vi "ReadXML_SRSI.vi"(8 "error in (no error)":errorcluster, 11 "XML File Path":path) -> (0 "error out":errorcluster, 2 "SRSI Parameters":T1={"sensitivity"=0.11032028469750889, "Filter"={"Tau (fs)"=9.75e-13, "fwhm (fs)"=3.2551150895140684e-13, "filter gaussian power"=30}, "Poly Fit Order"=4, "N XPW Loop"=3, "Scales Unit"=enum."nm", "Results average"=0, "Spectral filter"={"min"=0.0, "max"=0.0, "Level"=0.0}, "Apodization"={"Auto"=TRUE, "WL min"=6.000000000000001e-07, "WL max"=1.0000000000000002e-06}, "Warning levels"={"Min level"=5000.0, "Max level"=62000.0, "Min contrast"=0.1}, "NormXPW"=FALSE, "DisableChecks"=FALSE, "External\nFund. Spectrum"=FALSE, "XPW factors"={"Optimize"=enum."Never", "Blue Shift Correction"=0.0, "Parasite Amp"=0.0}}, 3 "XML File Path(duplicate)":path)   [LabVIEW 2020]
uses:
  SRSI_Parameters.ctl
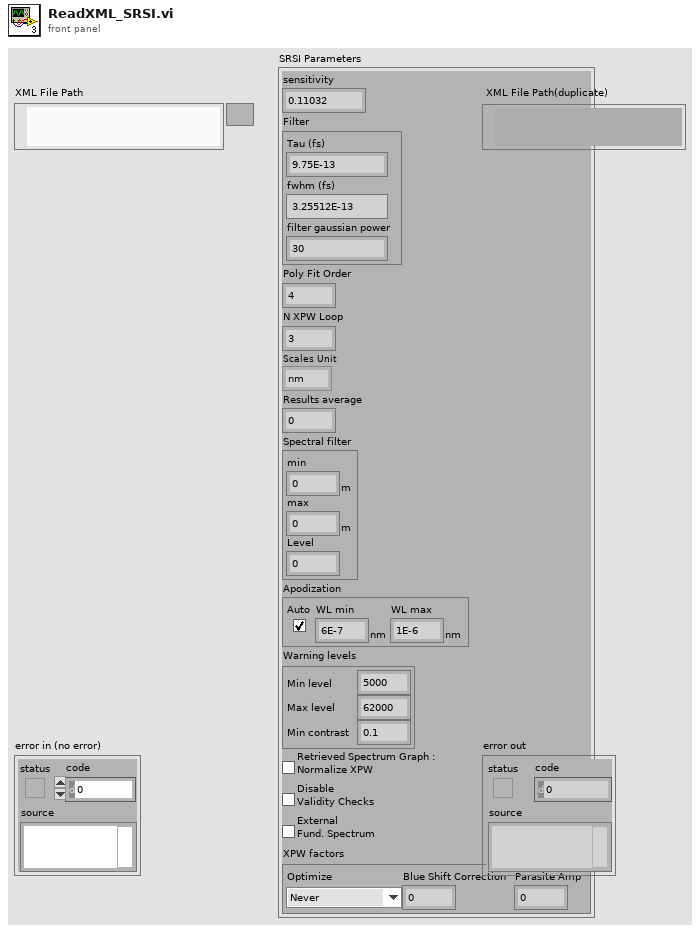
[diagram p1: front panel]
types:
  T1 = typedef "SRSI_Parameters.ctl" = cluster{"sensitivity":dbl, "Filter":cluster{"Tau (fs)":dbl[unit], "fwhm (fs)":dbl[unit], "filter gaussian power":i32}, "Poly Fit Order":i32, "N XPW Loop":u16, "Scales Unit":enum16{"nm", "THz", "cm^-1"}, "Results average":i32, "Spectral filter":cluster{"min":dbl[unit], "max":dbl[unit], "Level":dbl}, "Apodization":cluster{"Auto":bool, "WL min":dbl[unit], "WL max":dbl[unit]}, "Warning levels":cluster{"Min level":dbl, "Max level":dbl, "Min contrast":dbl}, "NormXPW":bool, "DisableChecks":bool, "External\nFund. Spectrum":bool, "XPW factors":cluster{"Optimize":enum16{"Never", "Once", "Ever"}, "Blue Shift Correction":dbl, "Parasite Amp":dbl}}
  T2 = enum16{"Get Variant Array From Measure", "Set Measure From Variant Array"}
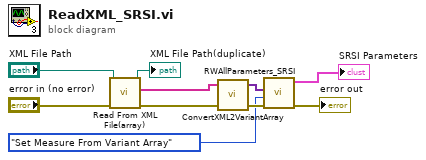
[diagram p0: block diagram]
diagram:
  n1 = call "Read From XML File(array).vi"("error in (no error)"="error in (no error)", "XML File Path"="XML File Path") -> ("error out"=w9:errorcluster, "XML Elements"=w10:string[], "XML File Path(duplicate)"=→"XML File Path(duplicate)":path)  [unwired: 7 in]
  n2 = call "ConvertXML2VariantArray.vi"("error in"=w9, "XML Strings"=w10) -> ("error out"=w8:errorcluster, "Variant Array"=w3:variant[])  [unwired: 2 in]
  n3 = call "RWAllParameters_SRSI.vi"("error in (no error)"=w8, "Read/Write"=T2."Set Measure From Variant Array", "Parameters In (Variant)"=w3) -> ("error out"=→"error out":errorcluster, "Parameters Out"=→"SRSI Parameters":T1)  [unwired: 6 in, 1 out]
